vi "NotifyMessages.vi"(6 "Add Alarm Button":bool=TRUE, 7 "milliseconds to wait":u32=8000, 8 "error in (no error)":errorcluster, 9 "Text 2":string="Baloon Tip Text", 10 "Icon (None) 2":i32(ring)=1 items=["None", "Info", "Warning", "Error"], 11 "Title 2":string="Balloon Tip") -> (0 "error out":errorcluster)   [LabVIEW 2020]
uses:
  <userlib>/TypeDefs/NotifyIcon Events.ctl
  <userlib>/TypeDefs/NotifyIcon Event Registration Actions.ctl
  <vilib>/Utility/error.llb/DialogType.ctl
  48bc6933-495b-478d-b49b-7395ee5d22cc.vi
  <vilib>/regexp/Match Regular Expression.xnode
panel:
  out "offset past match":i32
  out "message":string=" INSTRUCTIONS:\r\rNormal Use:  When using subVIs that incorporate the error in/error out (or error I/O) structure, place this handler where you want to inform the user of an error, typically at the end of the I/O data path, as the last action of the program.  If the error in error? is ERROR, the handler creates a message describing the error and its source.  If the type of dialog = 1 (default), the message is displayed to the user, who can only acknowedge it.  If the type = 2, the user can acknowledge the message or abort execution; aborting a program with active I/O is not recommended.  If the type = 0, no message is displayed; this is used to process the error programmatically, and the error out cluster elements are wired to individual terminals for that reason.  \r\rOther Use:\n\r\nlocal testing.  To test the error code of a subVI or function that does not have the error I/O structure, you can wire its error code and a source string to the local error code and error source inputs.  If error in error? indicates no error and error code is not equal to 0, the local code and source are substituted for the error in values, and error? is set TRUE (ERROR)."
  out "source out":string
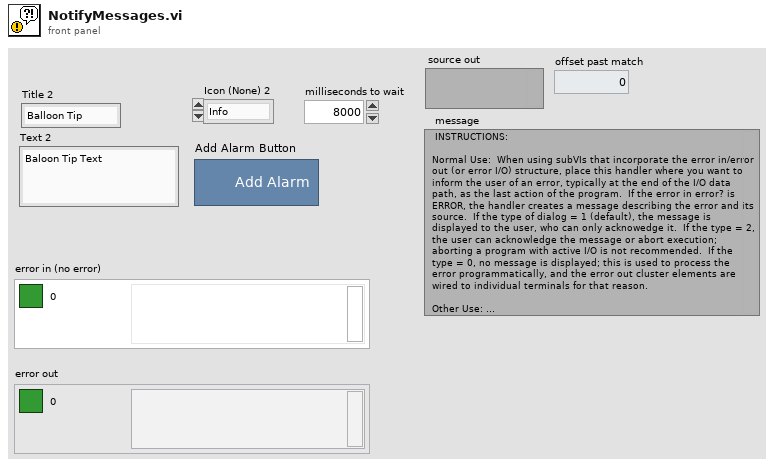
[diagram p1: front panel]
types:
  T1 = typedef "NotifyIcon Event Registration Actions.ctl" = enum16{"Initial Event Registration", "Add to Event Registration", "Destroy Events and Re-register"}
  T2 = typedef "NotifyIcon Events.ctl" = enum16{"BalloonTipClicked", "BalloonTipClosed", "BalloonTipShown", "Click", "Disposed", "DoubleClick", "MouseClick", "MouseDoubleClick", "MouseDown", "MouseMove", "MouseUp", "MenuItemClick", "MenuItemSelect"}
  T3 = typedef "DialogType.ctl" = u16
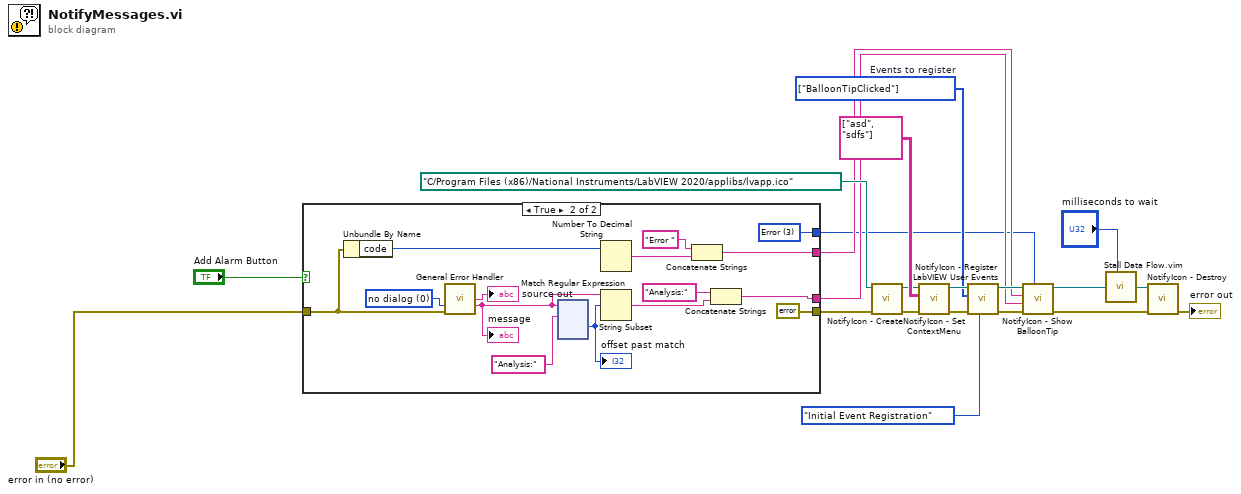
[diagram p0: block diagram]
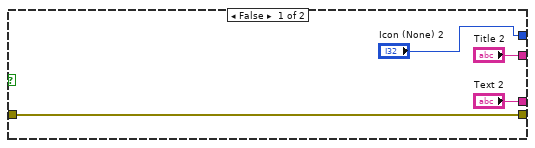
[diagram p2: hidden frame]
diagram:
  w14 = T2[] [enum."BalloonTipClicked"] items=["BalloonTipClicked", "BalloonTipClosed", "BalloonTipShown", "Click", "Disposed", "DoubleClick", "MouseClick", "MouseDoubleClick", "MouseDown", "MouseMove", "MouseUp", "MenuItemClick", "MenuItemSelect"]  # Events to register
  n1 = case shown="True" "Add Alarm Button" {
    tunnel: ["Text 2" w26] -> w10
    tunnel: ["Title 2" w36] -> w9
    tunnel: ["Icon (None) 2" w40] -> w8
    tunnel: [w22 errorcluster {"status"=FALSE, "code"=0, "source"=""} ("error in (no error)")] -> w5
    tunnel: "error in (no error)" -> [w22 w34]
    frame False {
    }
    frame True {
      w33 = T3 0 items=["no dialog", "OK message", "continue or stop message", "OK message + warnings", "continue/stop + warnings"] ("type of dialog (OK msg:1)")
      w40 = 3 items=["None", "Info", "Warning", "Error"] ("Icon (None) 3")
      n2 = Unbundle By Name(w34) -> ("code"=w38:i32)
      n3 = call <vilib>:"General Error Handler.vi"("type of dialog (OK msg:1)"=w33, "error in (no error)"=w34) -> ("source out"=→"source out":string, "message"=w30:string)  [unwired: 9 in, 3 out]
      "message" <- w30
      n4 = xnode "Match Regular Expression"("input string"=w30, "regular expression"="Analysis:") -> ("offset past match"=w29:i32)  [unwired: 4 in, 4 out]
      "offset past match" <- w29
      n5 = Number To Decimal String(number=w38) -> (decimal integer string=w37:string)  [unwired: 1 in]
      n6 = String Subset(string=w30, offset (0)=w29) -> (substring=w27:string)  [unwired: 1 in]
      n7 = Concatenate Strings("Error " ("string"), w37) -> (w36:string)
      n8 = Concatenate Strings("Analysis:" ("string"), w27) -> (w26:string)
    }
  }
  n9 = call <userlib>:"NotifyIcon - Create.vi"("error in"=w5, "Icon File Path"=path "C:/Program Files (x86)/National Instruments/LabVIEW 2020/applibs/lvapp.ico" ("Icon File Path 2")) -> ("error out"=w16:errorcluster, "NotifyIcon reference"=w18:refnum<k24>)  [unwired: 8 in]
  n10 = call <userlib>:"NotifyIcon - Set ContextMenu.vi"("error in"=w16, "Context Menu"=string[][] [["asd"], ["sdfs"]], "NotifyIcon reference in"=w18) -> ("error out"=w17:errorcluster, "NotifyIcon reference out"=w19:refnum<k24>)  [unwired: 7 in]
  n11 = call <userlib>:"NotifyIcon - Register LabVIEW User Events.vi"("Action"=NotifyIcon_Event_Registration_Actions."Initial Event Registration", "error in"=w17, "Events to register"=w14, "NotifyIcon reference in"=w19) -> ("error out"=w11:errorcluster, "NotifyIcon reference out"=w12:refnum<k24>)  [unwired: 5 in, 1 out]
  n12 = call <userlib>:"NotifyIcon - Show BalloonTip.vi"("Icon (None)"=w8, "error in"=w11, "Text"=w10, "Title"=w9, "NotifyIcon reference in"=w12) -> ("error out"=w7:errorcluster, "NotifyIcon reference out"=w4:refnum<k24>)  [unwired: 5 in]
  n13 = call "Stall Data Flow.vim"("value in"=w4, "milliseconds to wait"="milliseconds to wait") -> ("value out"=w3:refnum<k24>)  [unwired: 1 out]
  n14 = call <userlib>:"NotifyIcon - Destroy.vi"("error in"=w7, "NotifyIcon reference"=w3) -> ("error out"=→"error out":errorcluster)  [unwired: 9 in]
